vi "Test_PublicationLocked_RequestLock_ErrorReturned.vi"(8 "error in (no error)":errorcluster, 11 "TestMediator In":refnum<class "TestMediationSemantics.lvclass">) -> (0 "error out":errorcluster, 3 "TestMediator Out":refnum<class "TestMediationSemantics.lvclass">)   [LabVIEW 2020, in "TestMediationSemantics.lvclass"]
uses:
  TestMediationSemantics.lvclass
  TestMediationSemantics.lvclass/TestMediationSemantics.ctl
  Source/Mediator/Mediator/Mediator.lvclass
  <vilib>/ActorFramework/Actor/Actor.lvclass
  <vilib>/ActorFramework/Stop Msg/Stop Msg.lvclass
  Source/IMediator/IMediator Messages/Lock Publication Msg/Lock Publication Msg.lvclass
  modules/composed-transport/Source/Concrete/QueueTransport/QueueTransport.lvclass
  C:/Git/mva-core/Source/IMediator/IMediator/IMediator.lvclass
  C:/Program Files (x86)/National Instruments/LabVIEW 2020/vi.lib/ActorFramework/Actor/Actor.lvclass
  C:/Git/mva-core/Source/Mediator/Mediator/Mediator.lvclass
  C:/Git/mva-core/modules/composed-transport/Source/ITransport/ITransport.lvclass
  C:/Git/mva-core/modules/composed-transport/Source/Concrete/QueueTransport/QueueTransport.lvclass
panel:
  out "Lock Return Error":errorcluster
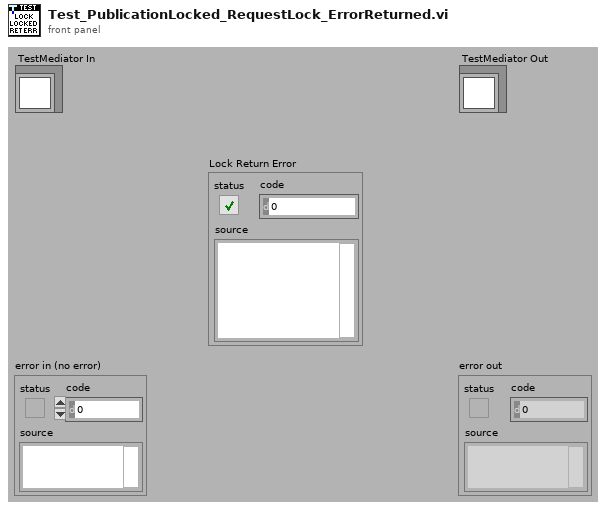
[diagram p1: front panel]
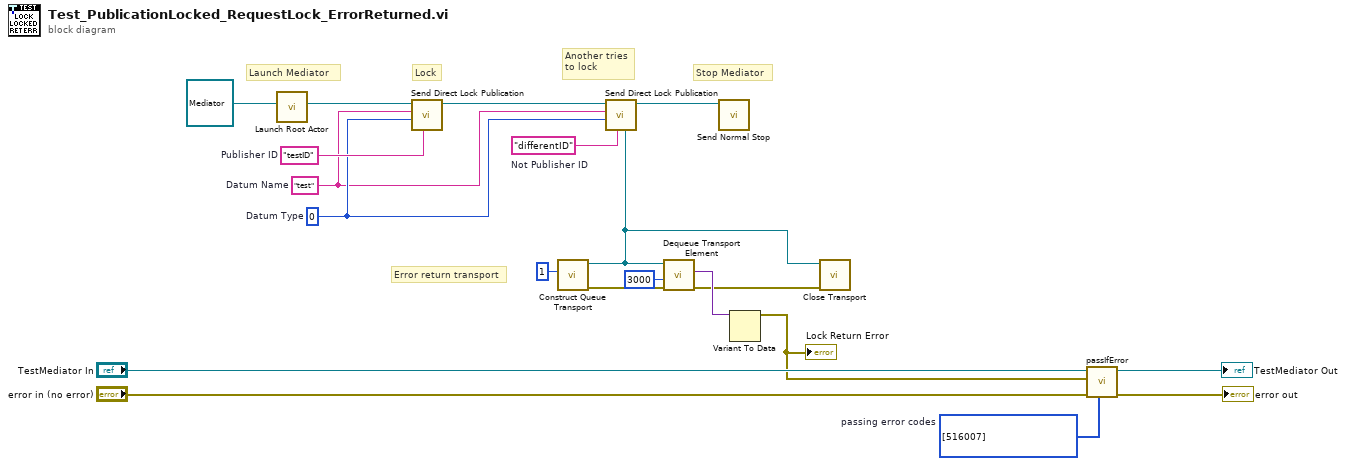
[diagram p0: block diagram]
diagram:
  w3 = i32[] [516007]  # passing error codes
  w8 = "differentID"  # Not Publisher ID
  w11 = "testID"  # Publisher ID
  w10 = 0  # Datum Type
  w9 = "test"  # Datum Name
  # "Error return transport"
  # "Lock"
  # "Launch Mediator"
  # "Stop Mediator"
  # "Another tries\nto lock"
  n1 = call <vilib>:"Launch Root Actor.vi"("Actor"=refnum<class "Mediator.lvclass"> refnum ("Mediator.lvlib:Mediator.lvclass")) -> ("Actor's Enqueuer"=w15:refnum<class "Message Enqueuer.lvclass">)  [unwired: 9 in, 1 out]
  n2 = call "Send Direct Lock Publication.vi"("Publisher ID"=w11, "Datum Type"=w10, "Datum Name"=w9, "Mediator Enqeuer"=w15) -> ("Mediator Enqueuer out"=w12:refnum<class "Message Enqueuer.lvclass">)  [unwired: 6 in, 1 out]
  n3 = call "Construct Queue Transport.vi"("Max Queue Size (-1)"=1) -> ("error out"=w6:errorcluster, "QueueTransport"=w2:refnum<class "QueueTransport.lvclass">)  [unwired: 9 in]
  n4 = call "Send Direct Lock Publication.vi"("Return Error Transport"=w2, "Publisher ID"=w8, "Datum Type"=w10, "Datum Name"=w9, "Mediator Enqeuer"=w12) -> ("Mediator Enqueuer out"=w7:refnum<class "Message Enqueuer.lvclass">)  [unwired: 5 in, 1 out]
  n5 = call "Dequeue Transport Element.vi"("error in (no error)"=w6, "Timeout In ms (-1)"=3000, "QueueTransport"=w2) -> ("error out"=w1:errorcluster, "Data"=w4:variant)  [unwired: 5 in, 2 out]
  n6 = call <vilib>:"Send Normal Stop.vi"("Message Enqueuer"=w7) -> ()  [unwired: 10 in, 1 out]
  n7 = Variant To Data(Variant=w4) -> (data=w5:errorcluster)  [unwired: 2 in, 1 out]
  "Lock Return Error" <- w5
  n8 = call-dynamic "Close Transport.vi"("error in (no error)"=w1, "QueueTransport"=w2) -> ()  [unwired: 9 in, 1 out]
  n9 = call-dynamic "passIfError.vi"("passing error codes (default = any error code)"=w3, "error in (no error)"="error in (no error)", "error"=w5, "TestCase in"="TestMediator In") -> ("error out"=→"error out":errorcluster, "TestCase out"=→"TestMediator Out":refnum<class "TestMediationSemantics.lvclass">)  [unwired: 6 in]
